vi "WeeklyTrends.vi"(8 "error in (no error)":errorcluster, 9 "AE-Groups":string[](array[string]), 10 "List of Weeks":u8[](array[numeric]), 11 "Report DVR in":refnum<data-value>) -> (0 "error out":errorcluster, 2 "SR Trends":string[][](array[string]))   [LabVIEW 2017, in "DS_Lib.lvlib" / "SRReportParser.lvlib"]
uses:
  SRReportParser.lvlib
  Modules/Private Controls/Report Data Cluster.ctl
  Modules/Private Controls/Data Raw.ctl
  Modules/Data Operations.lvlib
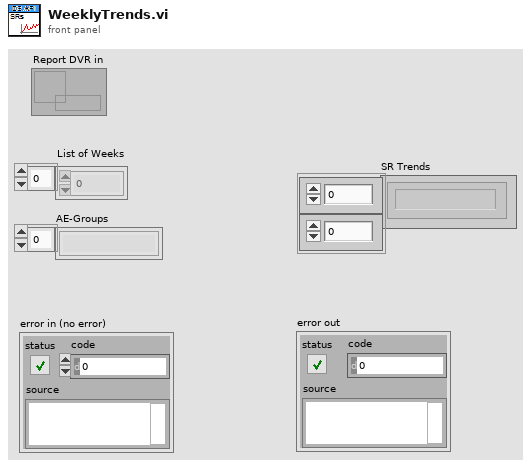
[diagram p1: front panel]
types:
  T1 = typedef "DS_Lib.lvlib/SRReportParser.lvlib/Weekly_SR_Stats.ctl" = cluster{"AE-Team":string, "In Work SRs":i32, "Open SRs":i32, "Solved within 5 WorkDays":i32, "Solved in more then 5 WorkDays":i32, "New SRs #":i32}
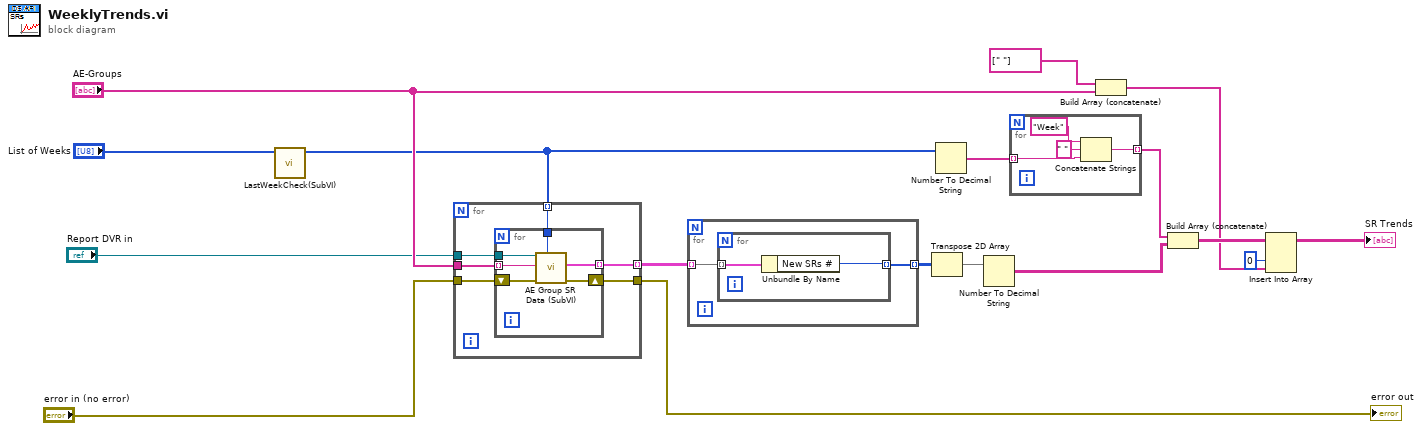
[diagram p0: block diagram]
diagram:
  n1 = call "LastWeekCheck(SubVI).vi"("List of Weeks"="List of Weeks") -> ("Array"=w2:u8[])  [unwired: 10 in]
  n2 = for {
    tunnel: [w23] -> w3 mode=indexing
    tunnel: w2 -> [w22] mode=indexing
    tunnel: "AE-Groups" -> [w21]
    tunnel: "error in (no error)" -> [w20]
    tunnel: [w19] -> w10
    tunnel: "Report DVR in" -> [w18]
    n3 = for {
      tunnel: [w29] -> w23 mode=indexing
      tunnel: w22 -> [w26]
      shift-right: [w28] -> w19
      shift-left: w20 -> [w27]
      tunnel: w21 -> [w25] mode=indexing
      tunnel: w18 -> [w24]
      n4 = call "AE Group SR Data (SubVI).vi"("Week"=w26, "error in (no error)"=w27, "AE-Group"=w25, "Report DVR in"=w24) -> ("error out"=w28:errorcluster, "Stats Out"=w29:T1)  [unwired: 6 in]
    }
  }
  "error out" <- w10
  n5 = for {
    tunnel: w3 -> [w31] mode=indexing
    tunnel: [w30] -> w4 mode=indexing
    n6 = for {
      tunnel: w31 -> [w33] mode=indexing
      tunnel: [w32] -> w30 mode=indexing
      n7 = Unbundle By Name(w33) -> ("New SRs #"=w32:i32)
    }
  }
  n8 = Transpose 2D Array(2D array=w4) -> (transposed array=w13:i32[][])
  n9 = Number To Decimal String(number=w2) -> (decimal integer string=w12:string[])  [unwired: 1 in]
  n10 = Number To Decimal String(number=w13) -> (decimal integer string=w14:string[][])  [unwired: 1 in]
  n11 = for {
    tunnel: w12 -> [w35] mode=indexing
    tunnel: [w34] -> w15 mode=indexing
    n12 = Concatenate Strings("Week" ("string"), " " ("string"), w35) -> (w34:string)
  }
  n13 = Build Array (concatenate)(string[] [" "] ("element"), "AE-Groups") -> (w8:string[])
  n14 = Build Array (concatenate)(w15, w14) -> (w16:string[][])
  n15 = Insert Into Array(array=w16, index (col)=0 ("disabled index (col)"), new element=w8) -> (→"SR Trends":string[][])  [unwired: 1 in]
